vi "Find sequences.vi"(11 "error in (no error)":errorcluster) -> (8 "Sequences":string[](array[string]), 15 "error out":errorcluster)   [LabVIEW 2011]
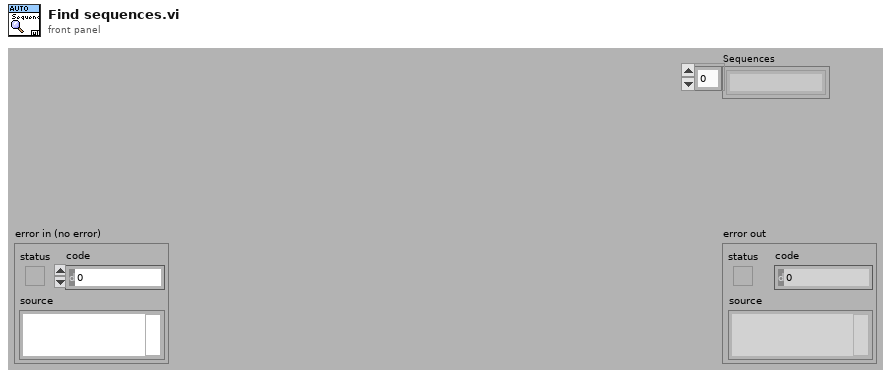
[diagram p1: front panel]
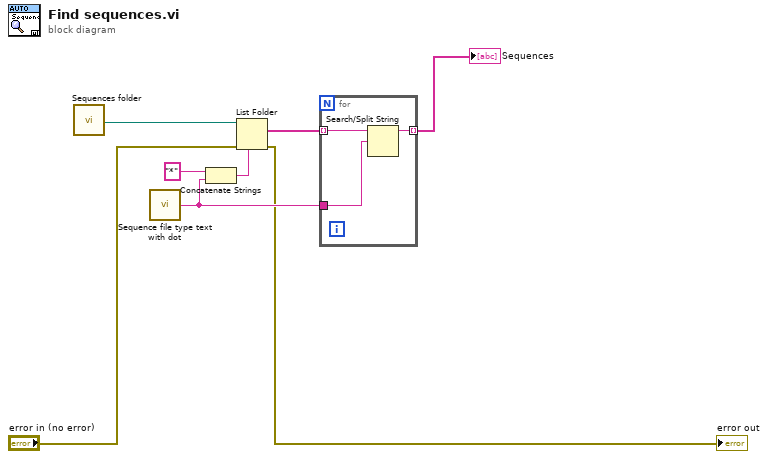
[diagram p0: block diagram]
diagram:
  n1 = call "Sequences folder.vi"() -> ("Sequence folder"=w8:path)  [unwired: 14 in, 1 out]
  n2 = call "Sequence file type text with dot.vi"() -> ("Sequrncefile type with dot"=w4:string)  [unwired: 14 in, 1 out]
  n3 = Concatenate Strings("*" ("string"), w4) -> (w7:string)
  n4 = List Folder(path=w8, pattern=w7, error in="error in (no error)") -> (filenames=w5:string[], error out=→"error out":errorcluster)  [unwired: 1 in, 2 out]
  n5 = for {
    tunnel: w5 -> [w11] mode=indexing
    tunnel: w4 -> [w10]
    tunnel: [w9] -> w3 mode=indexing
    n6 = Search/Split String(string=w11, search string/char (-)=w10) -> (substring before match=w9:string)  [unwired: 1 in, 2 out]
  }
  "Sequences" <- w3
